vi "ion_gauge_pressure.vi"() -> ()   [LabVIEW 2010]
doc: "The Basic Serial Read and Write example performs a Serial Port Read, a Serial Port Write, or a combination of these actions. The user selects the actions (read or write) on the front panel. If both are selected, the VI will write the data first, read data, and then close the VISA session that is opened to the port. This VI will wait until the specified number of bytes is received at the port. Only the number of bytes specified will be read.\n\nINSTRUCTIONS:\n1) Select the serial resource and configuration parameters (baud rate, data bits, parity, stop bits, flow control).\n2) Select the operations to be performed. \n3) Connect the serial port to your device. If no device is available, perform a loopback test by doing one of the following. Short pins 2 and 3 on a RS-232 cable or short pin 4 to pin 8 and pin 5 to pin 9 on a RS-485/422 cable. \n4) Run the VI to see the data read. (The \"read string\" will match the \"string to write\" if a loopback test was performed.)\n\nNote: The parameters set for the serial port must match the parameters of the connected instrument or device. In this example, the bytes to read parameter specifies the number of bytes that the serial port reads. If there were more bytes at the port than the number specified in bytes to read, those bytes would not be read. Also, if you specify to read more bytes than the number of bytes actually read, you might receive a timeout error message.\n\nOn the block diagram, the Configure Serial Port VI sets the configuration parameters. The front panel displays the controls used to configure the basic parameters, such as baud rate, data bits, and parity. Constants configure the other parameters the user probably does not need set. After the VISA Configure Serial Port VI opens the VISA session and configures the port, the VI passes the VISA resource name to other VIs that perform operations on that VISA resource. The VISA Write function sends a command to the serial device and the VISA Read function returns data based on the command. The VISA Close function then closes the reference to the serial device. It is important to close the reference; otherwise communication through with that port through protocols other than VISA might not be possible."
panel:
  in  "TC Pressure":bool caption="AC Pressure"
  out "TC Pressure (Torr)":dbl
  out "TC Pressure":cluster{dbl, dbl}[](graph)
  in  "AC Pressure":bool
  out "AC Pressure":cluster{dbl, dbl}[](graph)
  out "AC Pressure (Torr)":dbl
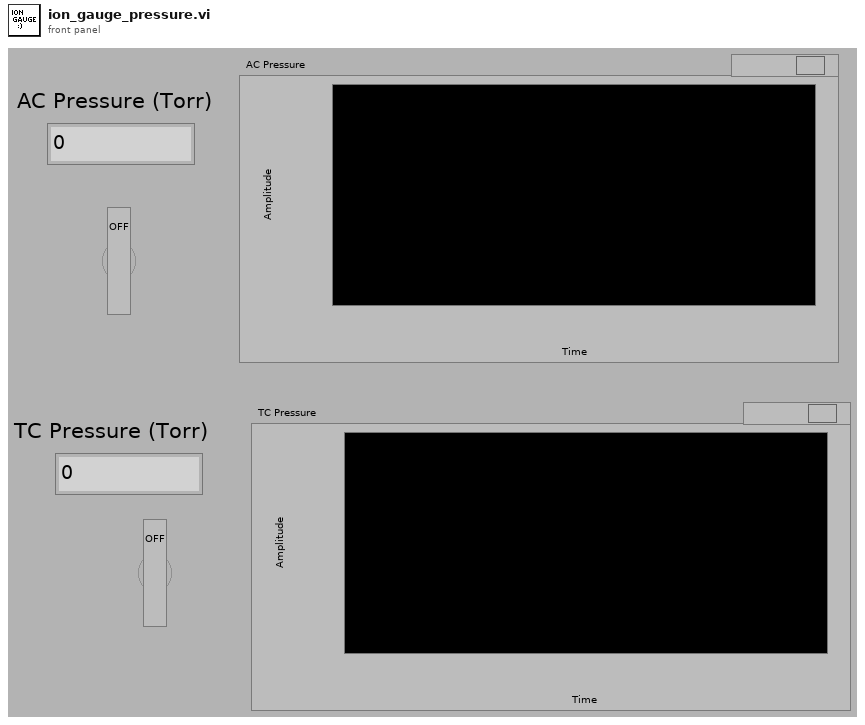
[diagram p1: front panel]
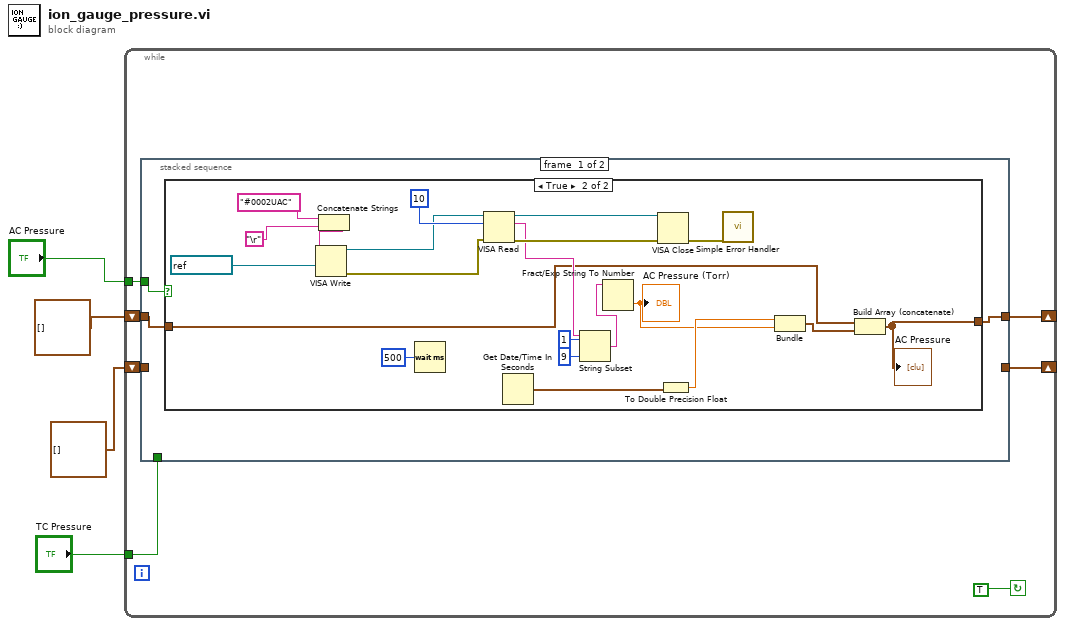
[diagram p0: block diagram]
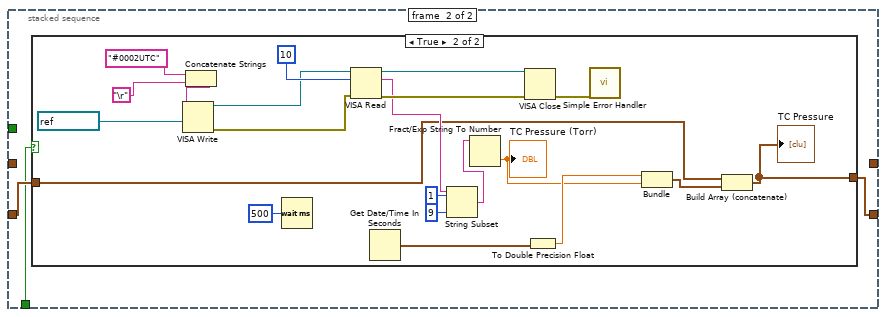
[diagram p3: hidden frame]
diagram:
  n1 = while {
    shift-right: [w5] -> _
    shift-left: cluster{dbl, dbl}[] [] -> [w11]
    tunnel: "AC Pressure" -> [w10]
    shift-right: [w7] -> _
    shift-left: cluster{dbl, dbl}[] [] -> [w8]
    tunnel: "TC Pressure" -> [w6]
    stop <- TRUE continue-if-true
    n2 = stacked-sequence {
      tunnel: w11 -> [w14 _]
      tunnel: w10 -> [w13 _]
      tunnel: w8 -> [_ w39]
      tunnel: [_ w38] -> w7
      tunnel: w6 -> [_ w37]
      tunnel: [w12 _] -> w5
      frame #0 {
        n3 = case shown="True" w13 {
          tunnel: w14 -> [w15 w19]
          tunnel: [w15 w16] -> w12
          frame False {
          }
          frame True {
            n4 = Concatenate Strings("#0002UAC" ("string"), "\r") -> (w34:string)
            n5 = VISA Write(VISA resource name=refnum<visa-resource-name> "COM4", write buffer=w34) -> (VISA resource name out=w29:refnum<visa-resource-name>, error out=w30:errorcluster)  [unwired: 1 in, 1 out]
            n6 = Wait (ms)(milliseconds to wait=u32 500) -> ()  [unwired: 1 out]
            n7 = VISA Read(VISA resource name=w29, byte count=u32 10 ("bytes to read 2"), error in (no error)=w30) -> (VISA resource name out=w28:refnum<visa-resource-name>, read buffer=w26:string, error out=w27:errorcluster)  [unwired: 1 out]
            n8 = Get Date/Time In Seconds() -> (seconds since 1Jan1904=w21:timestamp)
            n9 = String Subset(string=w26, offset (0)=1, length (rest)=9 ("length (rest)")) -> (substring=w24:string)
            n10 = Fract/Exp String To Number(string=w24) -> (number=w17:dbl)  [unwired: 3 in, 1 out]
            "AC Pressure (Torr)" <- w17
            n11 = VISA Close(VISA resource name=w28, error in (no error)=w27) -> (error out=w36:errorcluster)
            n12 = To Double Precision Float(number=w21) -> (double precision float=w18:dbl)
            n13 = call <vilib>:"Simple Error Handler.vi"("error in (no error)"=w36) -> ()  [unwired: 4 in, 5 out]
            n14 = Bundle(w18, w17) -> (w20:cluster{dbl, dbl})  [unwired: 1 in]
            n15 = Build Array (concatenate)(w19, w20) -> (w16:cluster{dbl, dbl}[])
            "AC Pressure" <- w16
          }
        }
      }
      frame #1 {
        n16 = case shown="True" w37 {
          tunnel: w39 -> [w40 w44]
          tunnel: [w40 w41] -> w38
          frame False {
          }
          frame True {
            n17 = Concatenate Strings("#0002UTC" ("string"), "\r") -> (w59:string)
            n18 = VISA Write(VISA resource name=refnum<visa-resource-name> "COM4", write buffer=w59) -> (VISA resource name out=w54:refnum<visa-resource-name>, error out=w55:errorcluster)  [unwired: 1 in, 1 out]
            n19 = Wait (ms)(milliseconds to wait=u32 500) -> ()  [unwired: 1 out]
            n20 = VISA Read(VISA resource name=w54, byte count=u32 10 ("bytes to read 2"), error in (no error)=w55) -> (VISA resource name out=w53:refnum<visa-resource-name>, read buffer=w51:string, error out=w52:errorcluster)  [unwired: 1 out]
            n21 = Get Date/Time In Seconds() -> (seconds since 1Jan1904=w46:timestamp)
            n22 = String Subset(string=w51, offset (0)=1, length (rest)=9 ("length (rest)")) -> (substring=w49:string)
            n23 = Fract/Exp String To Number(string=w49) -> (number=w42:dbl)  [unwired: 3 in, 1 out]
            "TC Pressure (Torr)" <- w42
            n24 = VISA Close(VISA resource name=w53, error in (no error)=w52) -> (error out=w61:errorcluster)
            n25 = To Double Precision Float(number=w46) -> (double precision float=w43:dbl)
            n26 = call <vilib>:"Simple Error Handler.vi"("error in (no error)"=w61) -> ()  [unwired: 4 in, 5 out]
            n27 = Bundle(w43, w42) -> (w45:cluster{dbl, dbl})  [unwired: 1 in]
            n28 = Build Array (concatenate)(w44, w45) -> (w41:cluster{dbl, dbl}[])
            "TC Pressure" <- w41
          }
        }
      }
    }
  }
